vi "substitute.vi"(6 "Error shown?":bool, 7 "Var value":dbl, 8 "Splitted string tokens":T1, 11 "Splitted string":T3) -> (0 "Tokens":T1, 3 "Substituted string":string[](array[string]), 4 "Was error?":bool)   [LabVIEW 2021]
uses:
  Controls/SplittedStringTokens.ctl
  Controls/Classes.ctl
  Controls/SplittedString.ctl
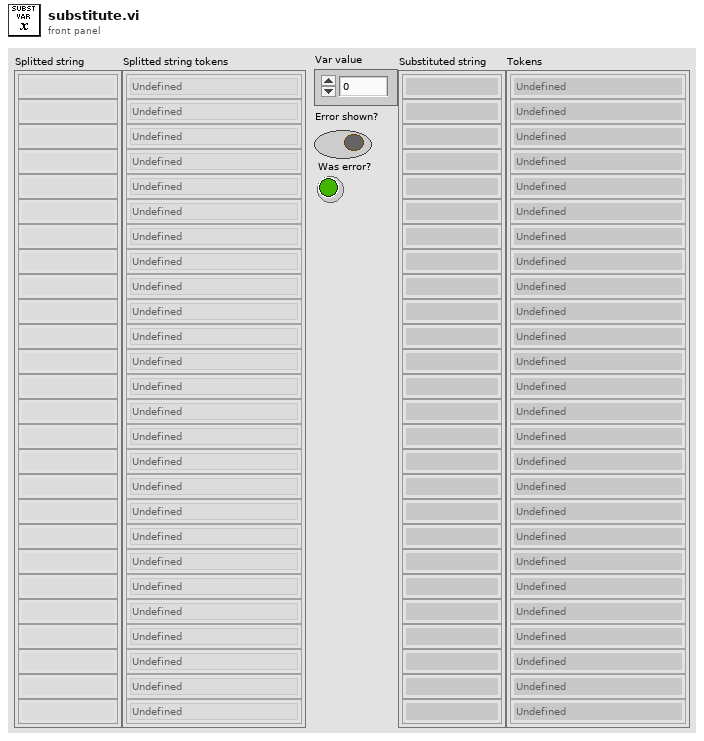
[diagram p1: front panel]
types:
  T1 = typedef "SplittedStringTokens.ctl" = T2[]
  T2 = typedef "Classes.ctl" = enum16{"Undefined", "Left paren", "Right paren", "Number", "Operator", "High level function", "Variable", "End of expression"}
  T3 = typedef "SplittedString.ctl" = string[]
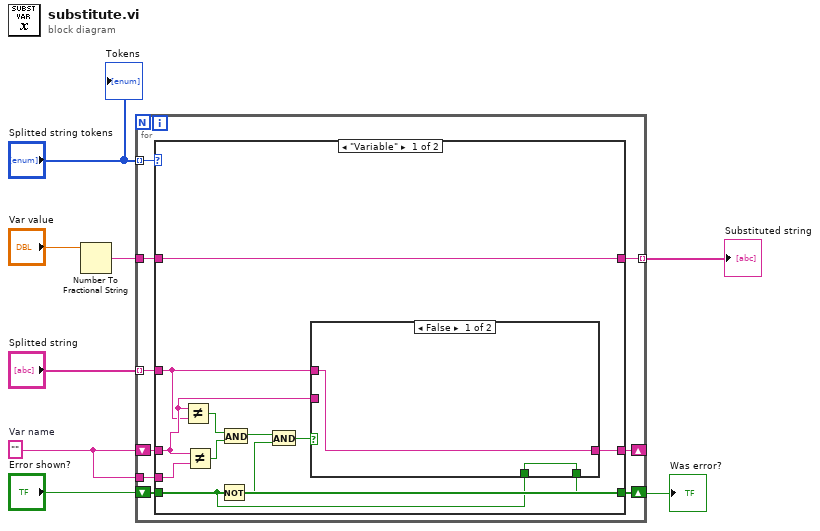
[diagram p0: block diagram]
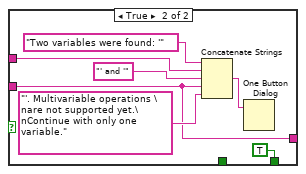
[diagram p2: hidden frame]
diagram:
  w7 = ""  # Var name
  n1 = Number To Fractional String(number="Var value") -> (F-format string=w5:string)  [unwired: 3 in]
  n2 = for {
    shift-right: [w15] -> _
    shift-left: w7 -> [w16]
    tunnel: "Splitted string tokens" -> [w17] mode=indexing
    tunnel: "Splitted string" -> [w14] mode=indexing
    tunnel: [w13] -> w4 mode=indexing
    tunnel: w7 -> [w12]
    tunnel: w5 -> [w11]
    shift-right: [w9] -> w1
    shift-left: "Error shown?" -> [w10]
    n3 = case shown="\"Variable\"" w17 {
      tunnel: w16 -> [w26 w41]
      tunnel: [w24 w41] -> w15
      tunnel: [w23 w40] -> w13
      tunnel: w14 -> [w25 w40]
      tunnel: w12 -> [w27 _]
      tunnel: w11 -> [w23 _]
      tunnel: w10 -> [w18 w39]
      tunnel: [w22 w39] -> w9
      frame "Variable" {
        n4 = Not Equal?(x=w26, y=w25) -> (x != y?=w28:bool)
        n5 = Not Equal?(x=w26, y=w27) -> (x != y?=w29:bool)
        n6 = Not(x=w18) -> (.not. x?=w21:bool)
        n7 = And(x=w28, y=w29) -> (x .and. y?=w19:bool)
        n8 = And(x=w19, y=w21) -> (x .and. y?=w20:bool)
        n9 = case shown="False" w20 {
          tunnel: w25 -> [w31 w34]
          tunnel: w26 -> [_ w33]
          tunnel: [w31 w33] -> w24
          tunnel: [w30 TRUE] -> w22
          tunnel: w18 -> [w30 _]
          frame False {
          }
          frame True {
            # "2 variables in the expression"
            n10 = Concatenate Strings("Two variables were found: '" ("string"), w34, "' and '" ("string"), w33, "'. Multivariable operations \nare not supported yet.\nContinue with only one variable." ("string")) -> (w38:string)
            n11 = One Button Dialog(message=w38) -> ()  [unwired: 1 in, 1 out]
          }
        }
      }
      frame Default {
      }
    }
  }
  "Substituted string" <- w4
  "Was error?" <- w1
  "Tokens" <- "Splitted string tokens"
